vi "Set Bleed-Fuel-ECS Cntrls.vi"(8 "error in (no error)":errorcluster, 11 "Bleed-Fuel-ECS Controls":T1 {"Bleed-Coarse-Knob" min=0.0 max=1000.0 step=1.0 scale=0.0..1000.0 scale format="%#.1g"; "Bleed-Fine-Knob" min=0.0 max=1000.0 step=1.0 scale=0.0..1000.0 scale format="%#.1g"}) -> (0 "error out":errorcluster)   [LabVIEW 2018, in "Outputs.lvlib"]
doc: "This subVI enqueues the named action in to the communications queue along with the input data."
uses:
  Outputs.lvlib
  Modules/Testing UI 1/Public Controls/Bleed-Fuel-ECS Controls.ctl
  Private Controls/Module Data.ctl
  Private Controls/Module Action.ctl
  Modules/Testing UI 1/Testing UI 1.lvlib
panel:
  # "Bleed Load Controls"
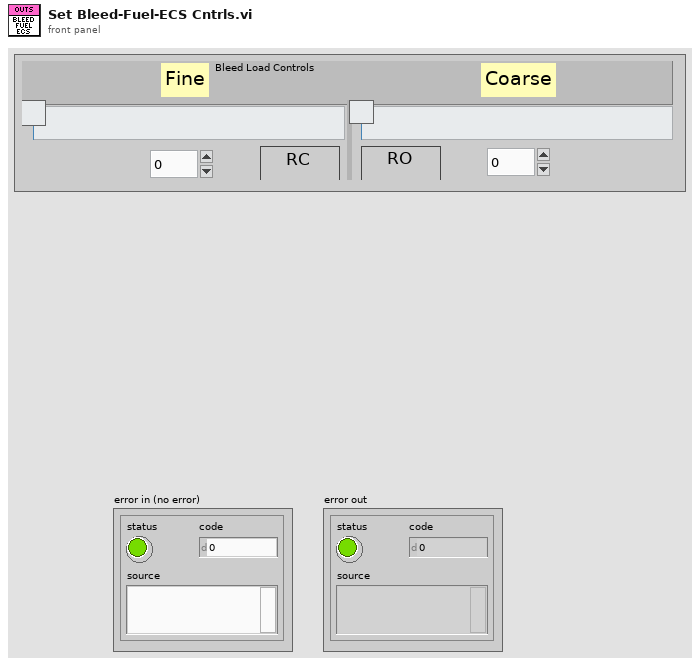
[diagram p1: front panel]
types:
  T1 = typedef "Testing UI 1.lvlib/Bleed-Fuel-ECS Controls.ctl" = cluster{"Coarse_RC":bool, "Coarse_RO":bool, "Bleed-Fine-Knob":dbl, "Bleed-Coarse-Knob":dbl}
  T2 = typedef "Outputs.lvlib/Module Data.ctl" = cluster{"Data":variant, "Action":T3}
  T3 = typedef "Outputs.lvlib/Module Action.ctl" = enum16{"Init", "Error", "Write 02-06-9265 Vals (AO)", "Write 02-01-9485 Vals (DO)", "Set APU&ECU Cntrls", "Set Bleed-Fuel-ECS Cntrls", "Set ECS Demnd Cluster", "Set Fuel Pres Regltr", "Write Single 02-00-9485 Chann", "Write Single 02-01-9485 Chann"}
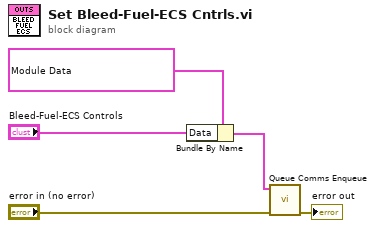
[diagram p0: block diagram]
diagram:
  n1 = Bundle By Name(cluster=T2 {"Data"=variant, "Action"=enum."Set Bleed-Fuel-ECS Cntrls"} ("element"), "Data"="Bleed-Fuel-ECS Controls") -> (w2:T2)
  n2 = call "Queue Comms Enqueue.vi"("error in (no error)"="error in (no error)", "element"=w2) -> ("error out"=→"error out":errorcluster)  [unwired: 9 in]
